vi "Devcon.Remove Device.vi"(8 "error in (no error)":errorcluster, 10 "DeviceID":string="USB\\VID_28DE&PID_2300&MI_02\\9&35BD5232&0&0002", 11 "DevconEXE":path=path "C:/Program Files (x86)/Windows Kits/10/Tools/x64/devcon") -> (0 "error out":errorcluster, 1 "StdOut":string, 2 "Cmd":string, 3 "Success":bool)   [LabVIEW 2018]
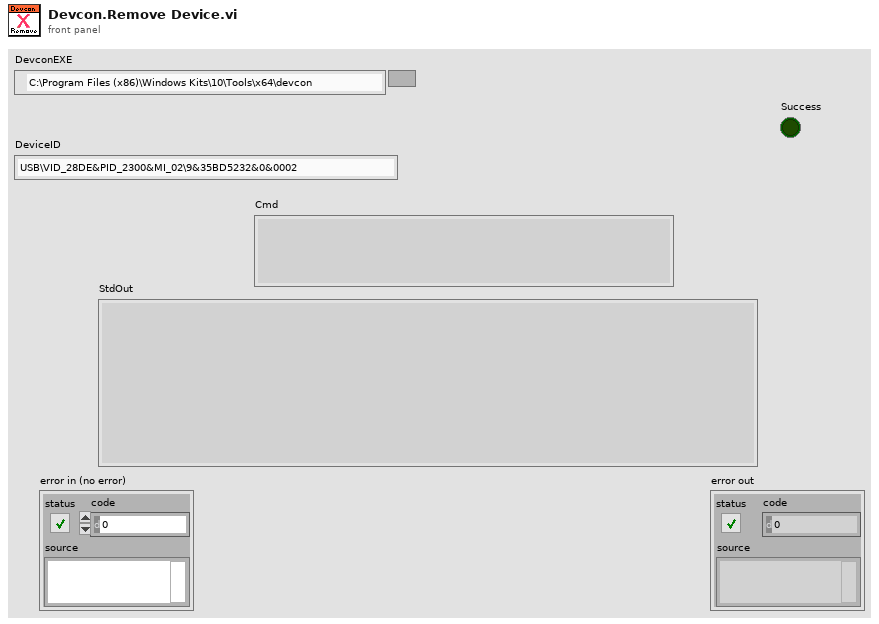
[diagram p1: front panel]
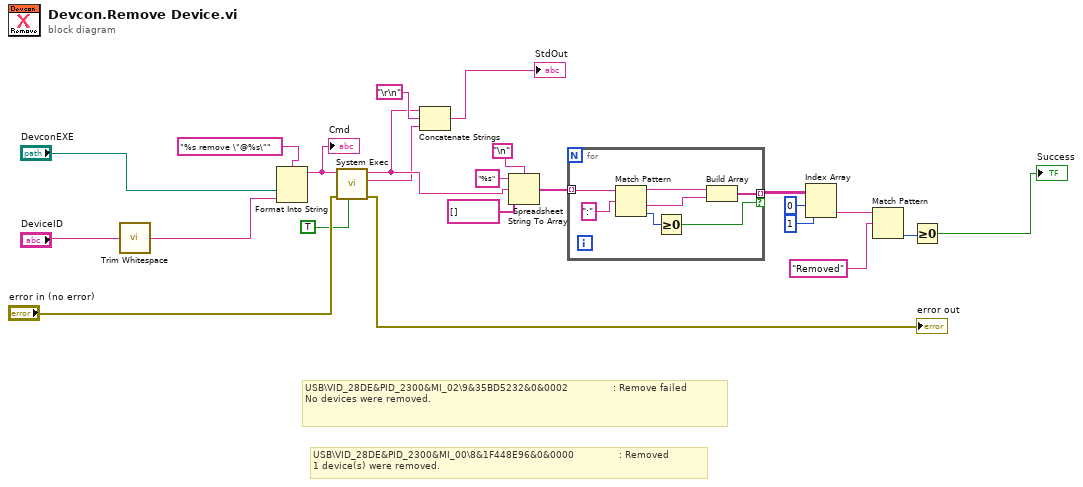
[diagram p0: block diagram]
diagram:
  # "USB\\VID_28DE&PID_2300&MI_00\\8&1F448E96&0&0000               : Removed\n1 device(s) were removed."
  # "USB\\VID_28DE&PID_2300&MI_02\\9&35BD5232&0&0002               : Remove failed\nNo devices were removed."
  n1 = call <vilib>:"Trim Whitespace.vi"("string"="DeviceID") -> ("trimmed string"=w5:string)  [unwired: 1 in]
  n2 = Format Into String(format string="%s remove \"@%s\"", "DevconEXE", w5) -> (resulting string=w22:string)  [unwired: 2 in, 1 out]
  "Cmd" <- w22
  n3 = call <vilib>:"System Exec.vi"("run minimized? (F)"=TRUE, "error in (no error)"="error in (no error)", "command line"=w22) -> ("error out"=→"error out":errorcluster, "standard error"=w2:string, "standard output"=w3:string)  [unwired: 5 in, 1 out]
  n4 = Concatenate Strings(w3, "\r\n", w2) -> (→"StdOut":string)
  n5 = Spreadsheet String To Array(delimiter (Tab)="\n", format string="%s", spreadsheet string=w3, array type (2D Dbl)=string[] [] ("Device List")) -> (array=w15:string[])
  n6 = for {
    tunnel: w15 -> [w30] mode=indexing
    tunnel: [w25] -> w14 mode=indexing if=w24
    n7 = Match Pattern(string=w30, regular expression=":") -> (before substring=w27:string, after substring=w26:string, offset past match=w28:i32)  [unwired: 1 in, 1 out]
    n8 = Greater Or Equal To 0?(x=w28) -> (x >= 0?=w24:bool)
    n9 = Build Array(w27, w26) -> (w25:string[])
  }
  n10 = Index Array(array=w14, index (row)=0, index (col)=1 ("disabled index (col)")) -> (element=w10:string)
  n11 = Match Pattern(string=w10, regular expression="Removed") -> (offset past match=w9:i32)  [unwired: 1 in, 3 out]
  n12 = Greater Or Equal To 0?(x=w9) -> (x >= 0?=→"Success":bool)
